vi "dfd_Validate Path.vi"(8 "error in (no error)":errorcluster, 11 "path in":path) -> (0 "error out":errorcluster, 3 "path out":path)   [LabVIEW 2017, in "NI_DigFilterLicensed.lvlib"]
uses:
  <vilib>/addons/Digital Filter Design/NI_DigFilterLicensed.lvlib
  <vilib>/addons/Digital Filter Design/_Misc.llb/dfd_Error Handlers (Single).vi
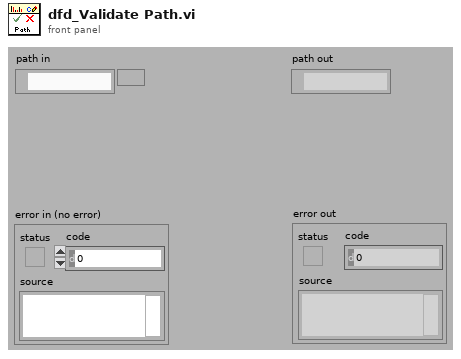
[diagram p1: front panel]
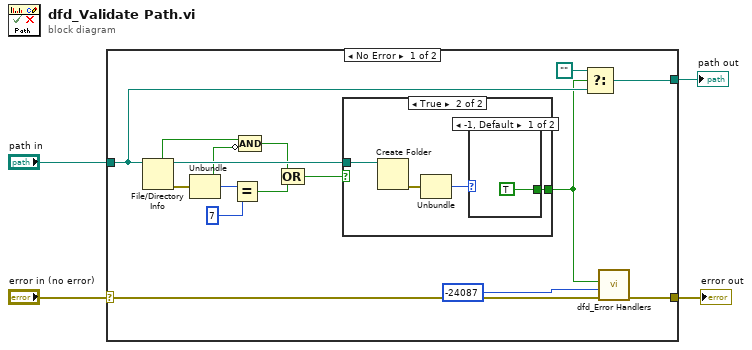
[diagram p0: block diagram]
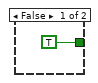
[diagram p2: hidden frame]
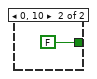
[diagram p3: hidden frame]
diagram:
  n1 = case shown="No Error" "error in (no error)" {
    selector: "error in (no error)" -> [w14 w28]
    tunnel: "path in" -> [w17 _]
    tunnel: [w16 _] -> w2
    tunnel: [w13 w28] -> w1
    frame No Error {
      n2 = File/Directory Info(path=w17) -> (path out=w19:path, directory=w9:bool, error out=w20:errorcluster)  [unwired: 1 in, 4 out]
      n3 = Unbundle(w20) -> ("status"=w8:bool, "code"=w11:i32)  [unwired: 1 out]
      n4 = Equal?(x=w11, y=7) -> (x = y?=w7:bool)
      n5 = Compound Arithmetic op=AND(w9, invert w8) -> (w6:bool)
      n6 = Compound Arithmetic op=OR(w6, w7) -> (w5:bool)
      n7 = case shown="True" w5 {
        tunnel: w19 -> [_ w25]
        tunnel: [TRUE w22] -> w15
        frame False {
        }
        frame True {
          n8 = Create Folder(path (use dialog)=w25) -> (error out=w24:errorcluster)  [unwired: 1 in, 3 out]
          n9 = Unbundle(w24) -> ("code"=w23:i32)  [unwired: 2 out]
          n10 = case shown="-1, Default" w23 {
            tunnel: [TRUE FALSE] -> w22
            frame -1, Default {
            }
            frame 0, 10 {
            }
          }
        }
      }
      n11 = Select(t=path "", s=w15, f=w17) -> (s? t:f=w16:path)
      n12 = call-poly <vilib>:"dfd_Error Handlers.vi"("error in (no error)"=w14, "error code"=-24087 ("ERR_INVALID_DIR"), "condition failed?"=w15) -> ("error out"=w13:errorcluster)  [unwired: 8 out]
    }
    frame Error {
    }
  }
  "path out" <- w2
  "error out" <- w1
